vi "BRig_Host__Loop_Producer__tcp_System__Data_prepareFilepaths.vi"(8 "input_arrFilenames":string[](array[string]), 9 "input_nFilenames":i32, 10 "input_storagePath":string, 11 "input_expPrefix":string) -> (0 "output_arrPath_target":path[](array[path]), 1 "output_arrPath_target_wExpPrefix":path[](array[path]), 2 "output_arrPath_source":path[](array[path]), 3 "output_arrPath_source_wExpPrefix":path[](array[path]))   [LabVIEW 2014]
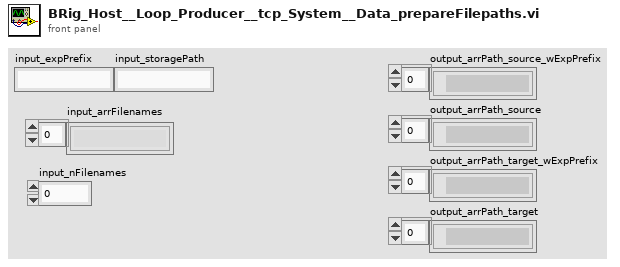
[diagram p1: front panel]
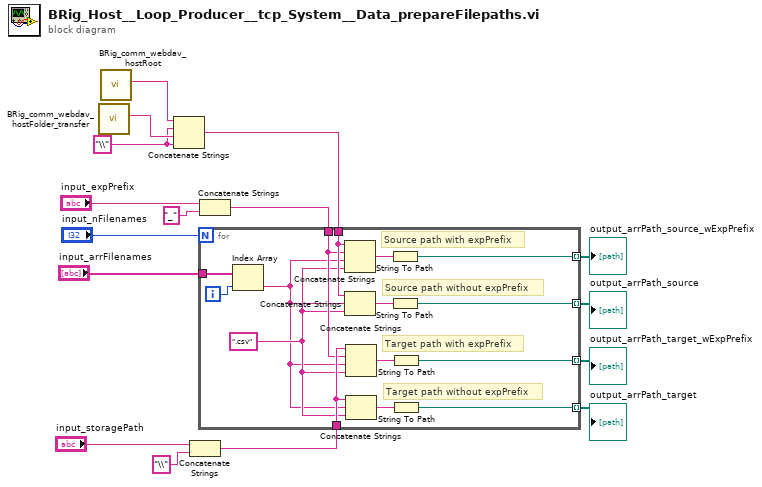
[diagram p0: block diagram]
diagram:
  w10 = "\\" ("string")
  n1 = call "BRig_comm_webdav_hostFolder_transfer.vi"() -> ("output_HostFolder"=w11:string)  [unwired: 11 in]
  n2 = call "BRig_comm_webdav_hostRoot.vi"() -> ("output_hostRoot"=w9:string)  [unwired: 11 in]
  n3 = Concatenate Strings(w9, w10, w11, w10) -> (w8:string)
  n4 = Concatenate Strings("input_storagePath", "\\" ("string")) -> (w5:string)
  n5 = Concatenate Strings("input_expPrefix", "_" ("string")) -> (w13:string)
  n6 = for {
    N: "input_nFilenames" -> [_]
    tunnel: w13 -> [w23]
    tunnel: "input_arrFilenames" -> [w31]
    tunnel: w8 -> [w27]
    tunnel: w5 -> [w24]
    tunnel: [w20] -> w4 mode=indexing
    tunnel: [w19] -> w3 mode=indexing
    tunnel: [w18] -> w2 mode=indexing
    tunnel: [w17] -> w1 mode=indexing
    i -> [w30]
    w22 = ".csv" ("string")
    # "Target path without expPrefix"
    # "Target path with expPrefix"
    # "Source path without expPrefix"
    # "Source path with expPrefix"
    n7 = Index Array(array=w31, index=w30) -> (element=w21:string)
    n8 = Concatenate Strings(w27, w23, w21, w22) -> (w29:string)
    n9 = Concatenate Strings(w27, w21, w22) -> (w28:string)
    n10 = Concatenate Strings(w24, w23, w21, w22) -> (w26:string)
    n11 = Concatenate Strings(w24, w21, w22) -> (w25:string)
    n12 = String To Path(string=w29) -> (path=w20:path)
    n13 = String To Path(string=w28) -> (path=w19:path)
    n14 = String To Path(string=w26) -> (path=w18:path)
    n15 = String To Path(string=w25) -> (path=w17:path)
  }
  "output_arrPath_source_wExpPrefix" <- w4
  "output_arrPath_source" <- w3
  "output_arrPath_target_wExpPrefix" <- w2
  "output_arrPath_target" <- w1
